vi "Set_Title_Button_NOk.vi"(8 "error in (no error)":errorcluster caption="entrée d'erreur (pas d'erreur)", 10 "Title_Button_NOk":string, 11 "Class Popup (Default) en entrée":refnum<class "Class Popup (Main).lvclass">) -> (0 "error out":errorcluster caption="sortie d'erreur", 3 "Class Popup (Default) en sortie":refnum<class "Class Popup (Main).lvclass">)   [LabVIEW 2020, in "Library Instrument & Equipement.lvlib" / "Library Popup.lvlib" / "Class Popup (Main).lvclass"]
uses:
  Class Popup (Main).lvclass
  Class Popup (Main).lvclass/Class Popup (Main).ctl
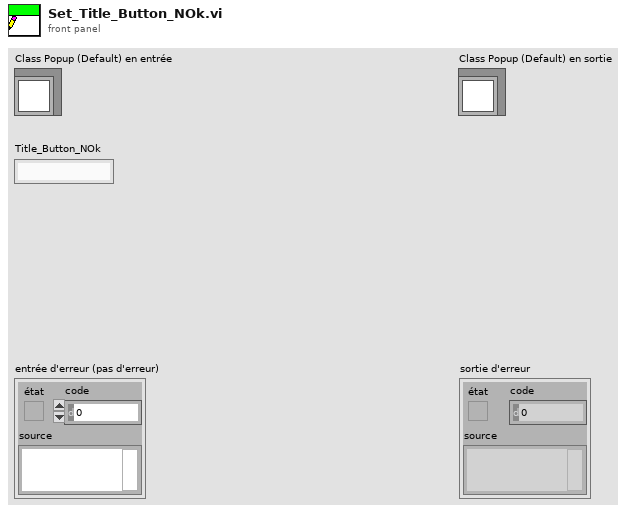
[diagram p1: front panel]
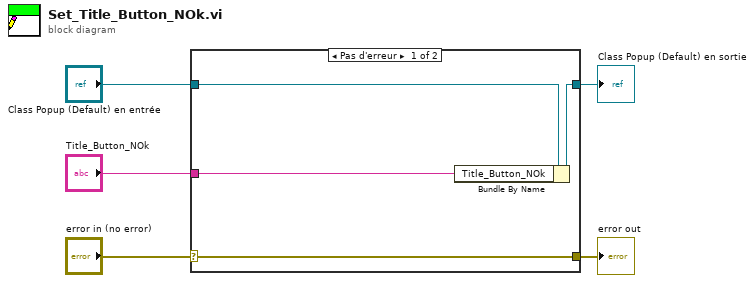
[diagram p0: block diagram]
diagram:
  n1 = case shown="Pas d'erreur" "error in (no error)" {
    selector: "error in (no error)" -> [w9 w10]
    tunnel: [w9 w10] -> w4
    tunnel: [w7 w11] -> w2
    tunnel: "Class Popup (Default) en entrée" -> [w8 w11]
    tunnel: "Title_Button_NOk" -> [w6 _]
    frame No Error {
      n2 = Bundle By Name(cluster=w8, "Title_Button_NOk"=w6) -> (w7:refnum<class "Class Popup (Main).lvclass">)
    }
    frame Error {
    }
  }
  "error out" <- w4
  "Class Popup (Default) en sortie" <- w2
